vi "Lab3_chirp_part1.vi"() -> ()   [LabVIEW 2010]
uses:
  <vilib>/Analysis/NI_AALBase.lvlib
  <vilib>/measure/NI_MABase.lvlib
  <vilib>/Analysis/NI_AALPro.lvlib
panel:
  out "Modulated Chirp":waveform(dbl)(graph)
  in  "Mod Index":dbl(slide) scale=0.0..1.0
  out "Chirp":dbl[](graph)
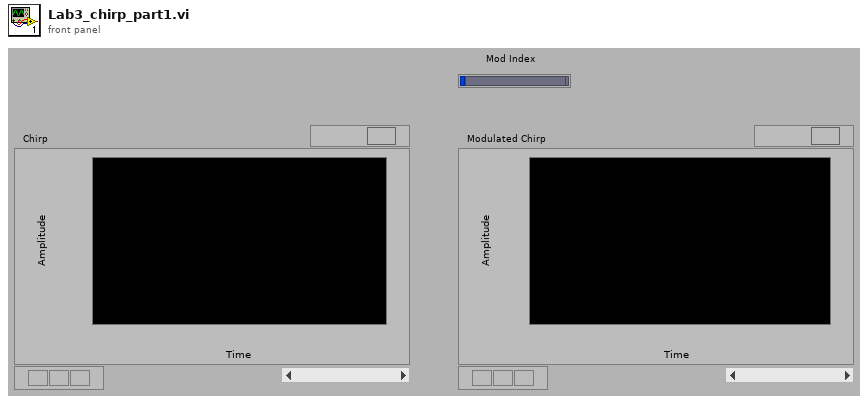
[diagram p1: front panel]
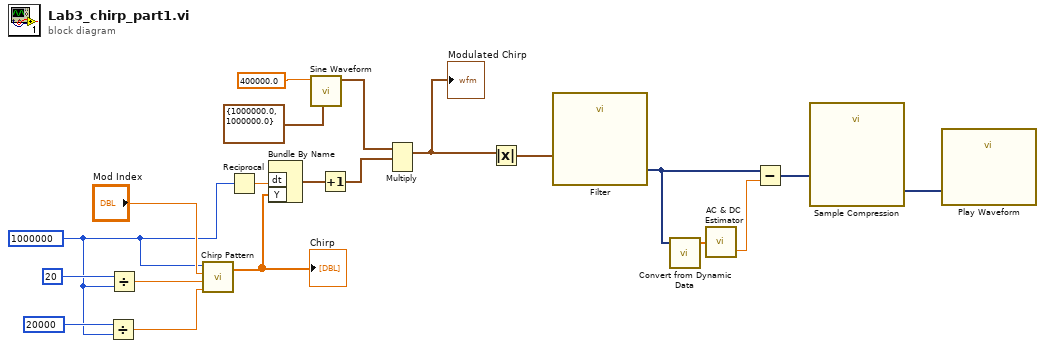
[diagram p0: block diagram]
diagram:
  w4 = 1000000 ("samples")
  n1 = Divide(x=20000 ("samples"), y=w4) -> (x/y=w18:dbl)
  n2 = Divide(x=20 ("samples"), y=w4) -> (x/y=w20:dbl)
  n3 = call <vilib>:"Chirp Pattern.vi"("f2"=w18, "f1"=w20, "amplitude"="Mod Index", "samples"=w4) -> ("Chirp Pattern"=w6:dbl[])  [unwired: 1 out]
  "Chirp" <- w6
  n4 = Reciprocal(x=w4) -> (1/x=w2:dbl)
  n5 = Bundle By Name("dt"=w2, "Y"=w6) -> (w7:waveform(dbl))  [unwired: 1 in]
  n6 = call <vilib>:"Sine Waveform.vi"("sampling info"=cluster{"Fs":dbl, "#s":dbl} {"Fs"=1000000.0, "#s"=1000000.0}, "frequency"=400000.0) -> ("signal out"=w15:waveform(dbl))  [unwired: 8 in, 1 out]
  n7 = Increment(x=w7) -> (x+1=w16:waveform(dbl))
  n8 = Multiply(1:w16, 2:w15) -> (0:w5:waveform(dbl))  [unwired: 1 in, 1 out]
  "Modulated Chirp" <- w5
  n9 = Absolute Value(x=w5) -> (abs(x)=w12:waveform(dbl))
  n10 = call "Filter"("Signal"=w12) -> ("Filtered Signal"=w10:dynamicdata)  [unwired: 9 in, 1 out]
  n11 = call "Convert from Dynamic Data"("Dynamic Data Type"=w10) -> ("Array"=w11:dbl[])  [unwired: 3 in]
  n12 = call <vilib>:"AC & DC Estimator.vi"("Signal (V)"=w11) -> ("DC estimate (V)"=w9:dbl)  [unwired: 1 out]
  n13 = Subtract(x=w10, y=w9) -> (x-y=w1:dynamicdata)
  n14 = call "Sample Compression"("Signals"=w1) -> ("Mean"=w3:dynamicdata)  [unwired: 8 in, 2 out]
  n15 = call "Play Waveform"("Data"=w3) -> ()  [unwired: 18 in, 1 out]
